vi "CH375_Reset.vi"(0 "Reset":bool) -> ()   [LabVIEW 2020]
uses:
  Global_CH375.vi
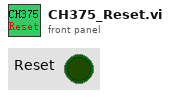
[diagram p1: front panel]
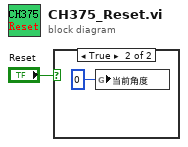
[diagram p0: block diagram]
diagram:
  n1 = case shown="True" "Reset" {
    frame False {
    }
    frame True {
      n2 = global write "Global_CH375.vi" "当前角度"(0) -> ()
    }
  }
